vi "Shifter Init.vi"(8 "Error in":errorcluster, 9 "Reverse Solenoid Channel":T1=enum."Solenoid 2", 10 "Forward Solenoid Channel":T1) -> (0 "Error Out":errorcluster)   [LabVIEW 2015]
uses:
  <vilib>/Rock Robotics/WPI/Solenoid/WPI_SolenoidChannel.ctl
  Support/Global Objects.vi
  <vilib>/Rock Robotics/WPI/Solenoid/WPI_SolenoidOpenDouble.vi
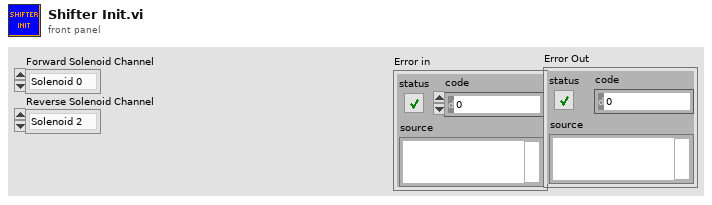
[diagram p1: front panel]
types:
  T1 = typedef "WPI_SolenoidChannel.ctl" = enum8{"Solenoid 0", "Solenoid 1", "Solenoid 2", "Solenoid 3", "Solenoid 4", "Solenoid 5", "Solenoid 6", "Solenoid 7", "Invalid"}
  T2 = typedef "Shifter.ctl" = cluster{"SolenoidDevRef":T3}
  T3 = typedef "WPI_SolenoidDevRef.ctl" = cluster{"DevStatus":errorcluster, "Pneumatics Control Module":u8, "Forward Solenoid Channel":T1, "Reverse Solenoid Channel":T1}
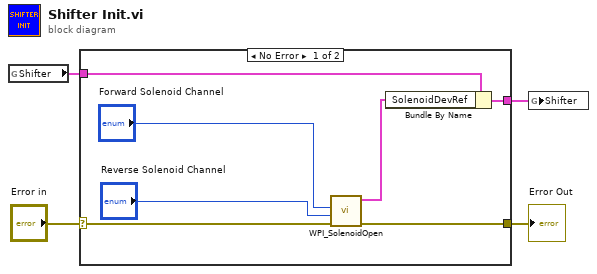
[diagram p0: block diagram]
diagram:
  n1 = global read "Global Objects.vi" "Shifter"() -> (w1:T2)
  n2 = case shown="No Error" "Error in" {
    selector: "Error in" -> [w9 w13]
    tunnel: [w8 w13] -> w3
    tunnel: [w6 w12] -> w2
    tunnel: w1 -> [w7 w12]
    frame No Error {
      n3 = call-poly <vilib>:"WPI_SolenoidOpen.vi"("error in (no error)"=w9, "Reverse Solenoid Channel"="Reverse Solenoid Channel", "Forward Solenoid Channel"="Forward Solenoid Channel") -> ("error out"=w8:errorcluster, "SolenoidDevRef"=w5:T3)  [unwired: 7 in]
      n4 = Bundle By Name(cluster=w7, "SolenoidDevRef"=w5) -> (w6:T2)
    }
    frame Error {
    }
  }
  "Error Out" <- w3
  n5 = global write "Global Objects.vi" "Shifter"(w2) -> ()
